vi "MDPtr ValidateFlattenToString.vi"() -> ()   [LabVIEW 2017]
uses:
  <vilib>/Utility/High Resolution Relative Seconds.vi
  <vilib>/measure/NI_MABase.lvlib
panel:
  out "length 2":i32
  out "length":i32
  out "Waveform Graph 5":waveform(dbl)(graph)
  out "Waveform Graph 4":waveform(dbl)(graph)
  out "x-y 2":u32
  out "Waveform Graph 3":dbl[](graph)
  out "Waveform Graph 2":i32[](graph)
  out "Waveform Graph":dbl[](graph)
  out "x-y":u32
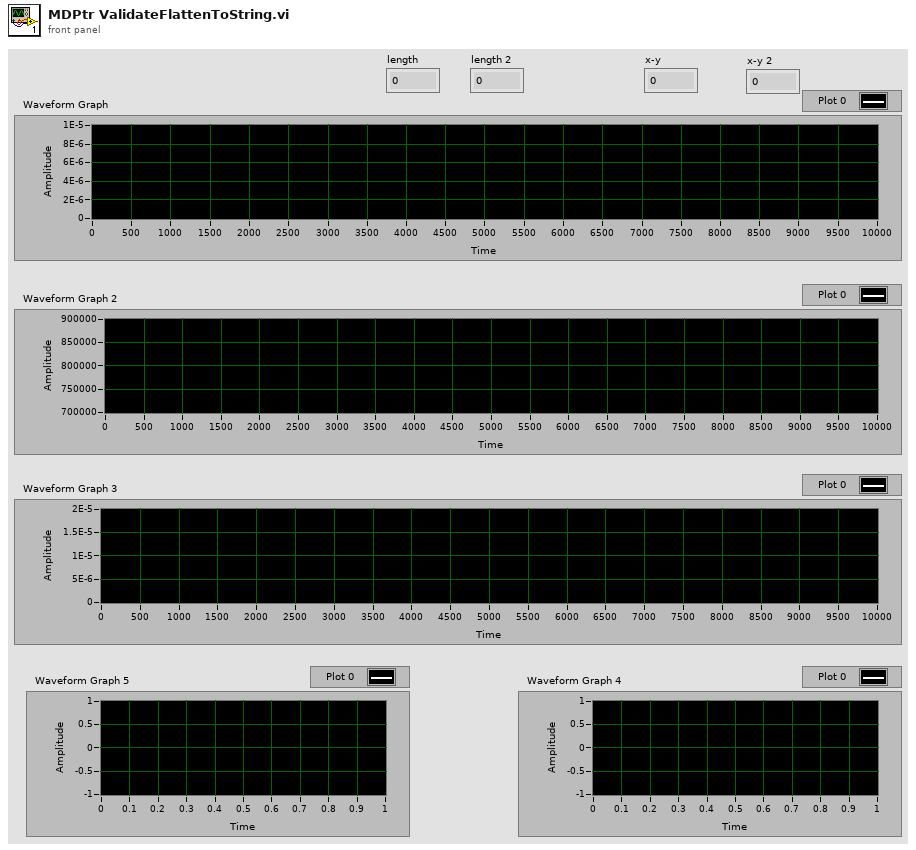
[diagram p1: front panel]
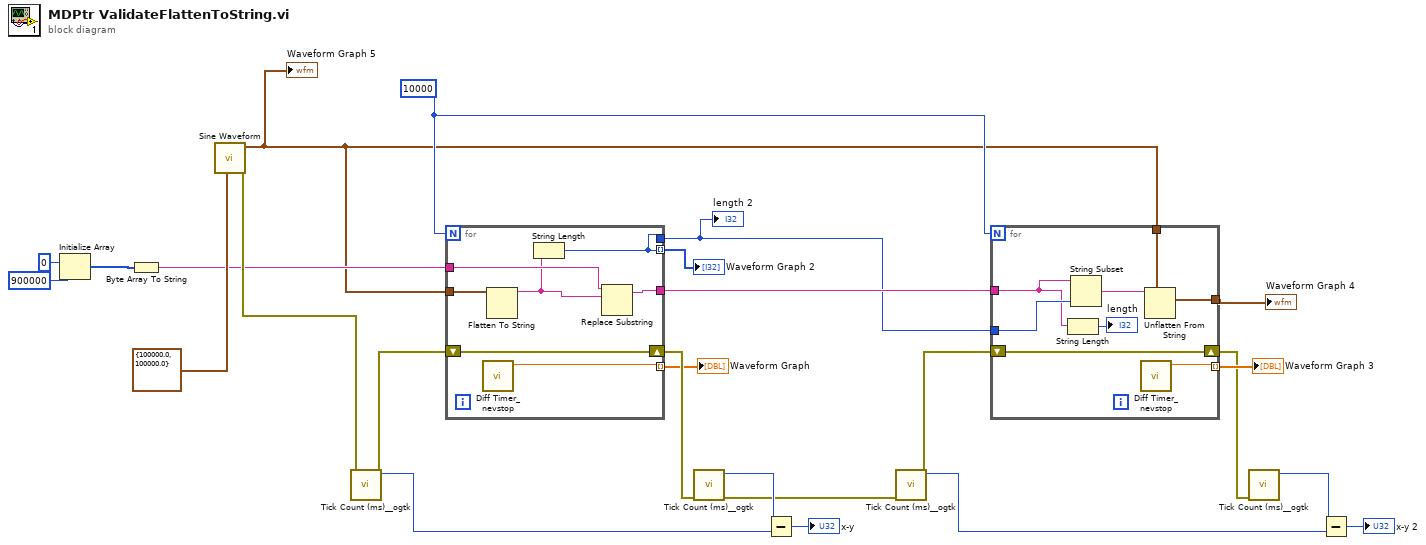
[diagram p0: block diagram]
diagram:
  w8 = 10000
  n1 = Initialize Array(u8 0 ("element"), 900000 ("dimension size")) -> (w5:u8[])
  n2 = Byte Array To String(unsigned byte array=w5) -> (string=w4:string)
  n3 = call <vilib>:"Sine Waveform.vi"("sampling info"=cluster{"Fs":dbl, "#s":dbl} {"Fs"=100000.0, "#s"=100000.0}) -> ("error out"=w22:errorcluster, "signal out"=w2:waveform(dbl))  [unwired: 9 in]
  "Waveform Graph 5" <- w2
  n4 = call <userlib>:"Tick Count (ms)__ogtk.vi"("error in (no error)"=w22) -> ("error out"=w21:errorcluster, "millisecond timer value"=w23:u32)  [unwired: 9 in]
  n5 = for {
    N: w8 -> [_]
    tunnel: w2 -> [w32]
    tunnel: [w31] -> w18 mode=indexing
    shift-right: [w30] -> w20
    shift-left: w21 -> [w30]
    tunnel: [w26] -> w17 mode=indexing
    tunnel: [w27] -> w9
    tunnel: [w26] -> w1
    tunnel: w4 -> [w29]
    n6 = call <userlib>:"Diff Timer_nevstop.vi"() -> ("time diff(s)"=w31:dbl)  [unwired: 10 in, 1 out]
    n7 = Flatten To String(anything=w32) -> (data string=w28:string)  [unwired: 3 in, 2 out]
    n8 = String Length(string=w28) -> (length=w26:i32)
    n9 = Replace Substring(4:w28, 5:w29) -> (1:w27:string)  [unwired: 2 in, 1 out]
  }
  "Waveform Graph" <- w18
  "Waveform Graph 2" <- w17
  "length 2" <- w1
  n10 = call <userlib>:"Tick Count (ms)__ogtk.vi"("error in (no error)"=w20) -> ("error out"=w10:errorcluster, "millisecond timer value"=w24:u32)  [unwired: 9 in]
  n11 = Subtract(x=w24, y=w23) -> (x-y=→"x-y":u32)
  n12 = call <userlib>:"Tick Count (ms)__ogtk.vi"("error in (no error)"=w10) -> ("error out"=w13:errorcluster, "millisecond timer value"=w12:u32)  [unwired: 9 in]
  n13 = for {
    N: w8 -> [_]
    tunnel: [w40] -> w16 mode=indexing
    shift-right: [w39] -> w14
    shift-left: w13 -> [w39]
    tunnel: w9 -> [w35]
    tunnel: w2 -> [w38]
    tunnel: [w37] -> w3
    tunnel: w1 -> [w36]
    n14 = String Length(string=w35) -> (length=→"length":i32)
    n15 = String Subset(string=w35, length (rest)=w36) -> (substring=w33:string)  [unwired: 1 in]
    n16 = call <userlib>:"Diff Timer_nevstop.vi"() -> ("time diff(s)"=w40:dbl)  [unwired: 10 in, 1 out]
    n17 = Unflatten From String(type=w38, binary string=w33) -> (value=w37:waveform(dbl))  [unwired: 3 in, 2 out]
  }
  "Waveform Graph 3" <- w16
  "Waveform Graph 4" <- w3
  n18 = call <userlib>:"Tick Count (ms)__ogtk.vi"("error in (no error)"=w14) -> ("millisecond timer value"=w11:u32)  [unwired: 9 in, 1 out]
  n19 = Subtract(x=w11, y=w12) -> (x-y=→"x-y 2":u32)
